vi "InitIntakeAndMagazine.vi"   [LabVIEW 2019]
uses:
  <vilib>/Rock Robotics/WPI/ThirdParty/Phoenix-LabVIEW/Motor Controller/Controls/CTRE_Phoenix_MotorControl_NeutralMode.ctl
  <vilib>/Rock Robotics/WPI/ThirdParty/REV Robotics/SPARK MAX/Typedef/Spark MAX Idle Mode.ctl
  <vilib>/Rock Robotics/WPI/Solenoid/WPI_SolenoidChannel.ctl
  refnums.vi
  <vilib>/Rock Robotics/WPI/Solenoid/WPI_SolenoidOpenDouble.vi
types:
  T1 = typedef "WPI_SolenoidChannel.ctl" = enum8{"Solenoid 0", "Solenoid 1", "Solenoid 2", "Solenoid 3", "Solenoid 4", "Solenoid 5", "Solenoid 6", "Solenoid 7", "Invalid"}
  T2 = typedef "Spark MAX Idle Mode.ctl" = enum16{"Coast", "Brake"}
  T3 = typedef "CTRE_Phoenix_MotorControl_NeutralMode.ctl" = enum8{"EEPROMSetting", "Override to Coast", "Override to Brake"}
  T4 = typedef "WPI_MotorControlDeviceRef.ctl" = cluster{"DeviceStatus":errorcluster, "Type":T5, "PWM":cluster{"PWM Channel":T6, "DeadBand":T7}, "CAN":cluster{"Device Number":u8, "SetOutput VI Ref":variant, "GetOutput VI Ref":variant, "Enable VI Ref":variant, "Disable VI Ref":variant, "Data":variant}, "Invert":bool, "DIO PWM":cluster{"PWM \"Enable\" Channel":T6, "DIOChannel":T8, "PWM Rate":dbl}}
  T5 = typedef "WPI_MotorControlType.ctl" = enum16{"PWM", "CAN", "DIO PWM"}
  T6 = typedef "FPGA_DIOPWMChannel.ctl" = enum8{"PWM 0", "PWM 1", "PWM 2", "PWM 3", "PWM 4", "PWM 5", "PWM 6", "PWM 7", "PWM 8", "PWM 9", "PWM MXP 0", "PWM MXP 1", "PWM MXP 2", "PWM MXP 3", "PWM MXP 4", "PWM MXP 5", "PWM MXP 6", "PWM MXP 7", "PWM MXP 8", "PWM MXP 9", "Invalid"}
  T7 = typedef "WPI_PWMDeadband.ctl" = cluster{"Name":string, "maxPositivePwm":i32, "minPositivePwm":i32, "centerPwm":i32, "maxNegativePwm":i32, "minNegativePwm":i32, "angularRange":u16}
  T8 = typedef "FPGA_DIOChannel.ctl" = enum8{"DIO 0", "DIO 1", "DIO 2", "DIO 3", "DIO 4", "DIO 5", "DIO 6", "DIO 7", "DIO 8", "DIO 9", "DIO MXP 0", "DIO MXP 1", "DIO MXP 2", "DIO MXP 3", "DIO MXP 4", "DIO MXP 5", "DIO MXP 6", "DIO MXP 7", "DIO MXP 8", "DIO MXP 9", "DIO MXP 10", "DIO MXP 11", "DIO MXP 12", "DIO MXP 13", "DIO MXP 14", "DIO MXP 15", "SPI Port CS1", "SPI Port CS2", "SPI Port CS3", "SPI Port MISO", "SPI Port MOSI", "Invalid"}
  T9 = typedef "WPI_SolenoidDevRef.ctl" = cluster{"DevStatus":errorcluster, "Pneumatics Control Module":u8, "Forward Solenoid Channel":T1, "Reverse Solenoid Channel":T1}
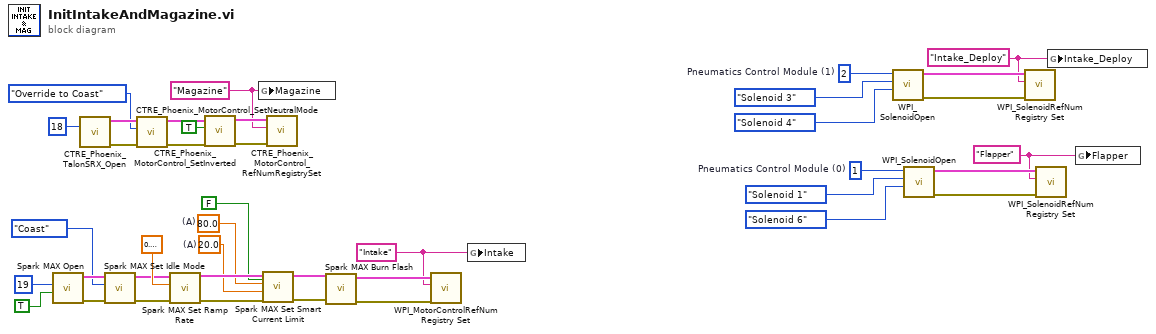
[diagram p0: block diagram]
diagram:
  w1 = "Flapper" ("refnum name")
  w6 = u8 1  # Pneumatics Control Module (0)
  w7 = "Intake_Deploy" ("refnum name")
  w12 = u8 2  # Pneumatics Control Module (1)
  w19 = 80.0  # (A)
  w18 = 20.0  # (A)
  w15 = "Intake" ("refnum name")
  w31 = "Magazine" ("refnum name")
  n1 = call <vilib>:"Spark MAX Open.vi"("Invert"=TRUE, "Device Number"=u8 19 ("Drive 1R")) -> ("error out"=w26:errorcluster, "MotorControlDeviceRef"=w29:T4)  [unwired: 8 in]
  n2 = call <vilib>:"CTRE_Phoenix_TalonSRX_Open.vi"("Device Number"=u8 18) -> ("error out"=w40:errorcluster, "CAN Talon SRX Ref"=w39:T4)  [unwired: 9 in]
  n3 = call <vilib>:"Spark MAX Set Idle Mode.vi"("error in (no error)"=w26, "Idle Mode"=Spark_MAX_Idle_Mode."Coast", "MotorControlDeviceRef in"=w29) -> ("error out"=w13:errorcluster, "MotorControlDeviceRef out"=w14:T4)  [unwired: 7 in]
  n4 = call <vilib>:"CTRE_Phoenix_MotorControl_SetNeutralMode.vi"("error in (no error)"=w40, "Motor Control Neutral Mode"=CTRE_Phoenix_MotorControl_NeutralMode."Override to Coast", "PhoenixMotorControlDevRef"=w39) -> ("error out"=w38:errorcluster, "PhoenixMotorControlDevRef"=w37:T4)  [unwired: 7 in]
  n5 = call <vilib>:"Spark MAX Set Ramp Rate.vi"("error in (no error)"=w13, "Seconds from neutral to full (0)"=sgl 0.2, "MotorControlDeviceRef in"=w14) -> ("error out"=w23:errorcluster, "MotorControlDeviceRef"=w20:T4)  [unwired: 7 in]
  n6 = call <vilib>:"CTRE_Phoenix_MotorControl_SetInverted.vi"("error in (no error)"=w38, "Invert?"=TRUE, "PhoenixMotorControlDevRef"=w37) -> ("error out"=w35:errorcluster, "PhoenixMotorControlDevRef"=w36:T4)  [unwired: 7 in]
  n7 = global write "refnums.vi" "Magazine"(w31) -> ()
  n8 = call <vilib>:"Spark MAX Set Smart Current Limit.vi"("Linearized Limit Enabled (F)"=FALSE, "error in (no error)"=w23, "Free Speed Current Limit (20A)"=w18, "Primay Current Limit (80A)"=w19, "MotorControlDeviceRef in"=w20) -> ("error out"=w22:errorcluster, "MotorControlDeviceRef out"=w21:T4)  [unwired: 5 in]
  n9 = call <vilib>:"CTRE_Phoenix_MotorControl_RefNumRegistrySet.vi"("error in (no error)"=w35, "refnum name"=w31, "PhoenixMotorControlDevRef"=w36) -> ()  [unwired: 7 in, 2 out]
  n10 = call <vilib>:"Spark MAX Burn Flash.vi"("error in"=w22, "MotorControlDeviceRef"=w21) -> ("error out"=w24:errorcluster, "MotorControlDeviceRef"=w25:T4)  [unwired: 8 in]
  n11 = call <vilib>:"WPI_MotorControlRefNum Registry Set.vi"("error in (no error)"=w24, "refnum name"=w15, "MotorControlDevRef"=w25) -> ()  [unwired: 7 in, 2 out]
  n12 = global write "refnums.vi" "Intake"(w15) -> ()
  n13 = call-poly <vilib>:"WPI_SolenoidOpen.vi"("Reverse Solenoid Channel"=WPI_SolenoidChannel."Solenoid 4", "Forward Solenoid Channel"=WPI_SolenoidChannel."Solenoid 3", "Pneumatics Control Module (0)"=w12) -> ("error out"=w8:errorcluster, "SolenoidDevRef"=w9:T9)  [unwired: 7 in]
  n14 = call-poly <vilib>:"WPI_SolenoidOpen.vi"("Reverse Solenoid Channel"=WPI_SolenoidChannel."Solenoid 6", "Forward Solenoid Channel"=WPI_SolenoidChannel."Solenoid 1", "Pneumatics Control Module (0)"=w6) -> ("error out"=w2:errorcluster, "SolenoidDevRef"=w3:T9)  [unwired: 7 in]
  n15 = call <vilib>:"WPI_SolenoidRefNum Registry Set.vi"("error in (no error)"=w8, "refnum name"=w7, "SolenoidDevRef"=w9) -> ()  [unwired: 7 in, 2 out]
  n16 = call <vilib>:"WPI_SolenoidRefNum Registry Set.vi"("error in (no error)"=w2, "refnum name"=w1, "SolenoidDevRef"=w3) -> ()  [unwired: 7 in, 2 out]
  n17 = global write "refnums.vi" "Intake_Deploy"(w7) -> ()
  n18 = global write "refnums.vi" "Flapper"(w1) -> ()
